vi "XYZ-field_to_current.vi"(0 "X":dbl, 1 "Y":dbl, 2 "Z":dbl) -> (3 "current 1":dbl, 4 "current 2":dbl, 5 "current 3":dbl, 6 "current 4":dbl)   [LabVIEW 2011]
uses:
  <vilib>/silver_ctls/ArrayMatrixCluster/Real Matrix NI_Silver.ctl
  <vilib>/Analysis/Matrix/Numeric/Conversions/Array To Matrix - RA.vi
  <vilib>/Analysis/7linalg.llb/Solve Linear Equations (multiple right hand).vi
  <vilib>/Analysis/Matrix/Numeric/Conversions/Matrix To Array - RM.vi
  <vilib>/Analysis/NI_AALPro.lvlib
  <vilib>/Analysis/Matrix/NI_Matrix.lvlib
panel:
  out "error":i32
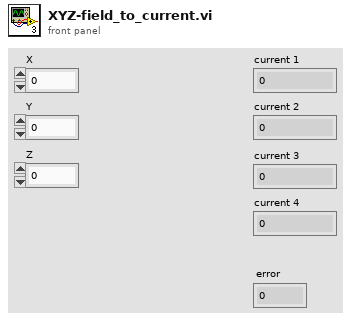
[diagram p1: front panel]
types:
  T1 = typedef "Real Matrix NI_Silver.ctl" = dbl[][]
  T2 = typedef "NI_Matrix.lvlib/RealMatrix.ctl" = dbl[][]
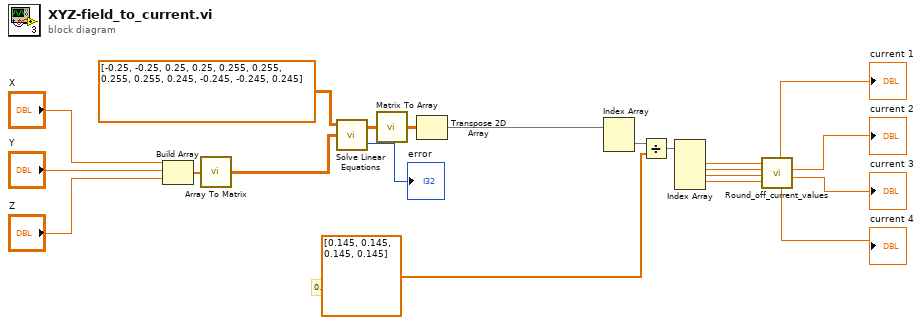
[diagram p0: block diagram]
diagram:
  # "0.145"
  n1 = Build Array("X", "Y", "Z") -> (w20:dbl[])
  n2 = call-poly <vilib>:"Array To Matrix.vi"("Real 1D Array"=w20) -> ("Real Matrix (Column Vector)"=w19:T2)
  n3 = call-poly <vilib>:"Solve Linear Equations.vi"("Known Matrix"=w19, "Input Matrix"=T1 [[-0.25, -0.25, 0.25, 0.25], [0.255, 0.255, 0.255, 0.255], [0.245, -0.245, -0.245, 0.245]] ("Real Matrix")) -> ("error"=→"error":i32, "Solution Matrix"=w18:T2)  [unwired: 1 in]
  n4 = call-poly <vilib>:"Matrix To Array.vi"("Real Matrix"=w18) -> ("Real 2D Array"=w17:dbl[][])
  n5 = Transpose 2D Array(2D array=w17) -> (transposed array=w15:dbl[][])
  n6 = Index Array(array=w15) -> (element=w16:dbl[])  [unwired: 2 in]
  n7 = Divide(x=w16, y=dbl[] [0.145, 0.145, 0.145, 0.145]) -> (x/y=w14:dbl[])
  n8 = Index Array(array=w14) -> (element #1=w13:dbl, element #2=w12:dbl, element #3=w11:dbl, element #4=w10:dbl)  [unwired: 4 in]
  n9 = call "Round_off_current_values.vi"("Numeric 4"=w10, "Numeric 3"=w11, "Numeric 2"=w12, "Numeric"=w13) -> ("Current 3"=→"current 3":dbl, "Current 2"=→"current 2":dbl, "Current 1"=→"current 1":dbl, "Current 4"=→"current 4":dbl)  [unwired: 4 in]
